vi "VIE.Module.Queued Message Handler.destroy.QueuedMessageHandler.vi"(8 "error in (no error)":errorcluster, 10 "QueuedMessageHandler.dqGOOPClass (in)":T1) -> (0 "error out":errorcluster)   [LabVIEW 2010, in "VIE.Module.Queued Message Handler.QueuedMessageHandler.dqGOOPClass.lvlib"]
uses:
  VIE.Module.Queued Message Handler.QueuedMessageHandler.dqGOOPClass.lvlib
  VIE.Module.Queued Message Handler.dqClass_ObjectReference.ctl
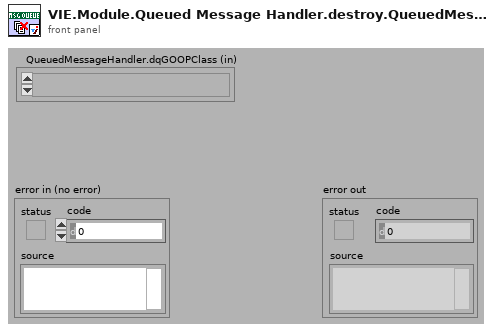
[diagram p1: front panel]
types:
  T1 = typedef "VIE.Module.Queued Message Handler.QueuedMessageHandler.dqGOOPClass.lvlib/VIE.Module.Queued Message Handler.dqClass_ObjectReference.ctl" = refnum<k1>
  T2 = typedef "VIE.Module.Queued Message Handler.QueuedMessageHandler.dqGOOPClass.lvlib/VIE.Module.Queued Message Handler.dqClass_ObjectData.ctl" = cluster{"Message Queue":refnum<queue>, "Log File Refnum":refnum<file>}
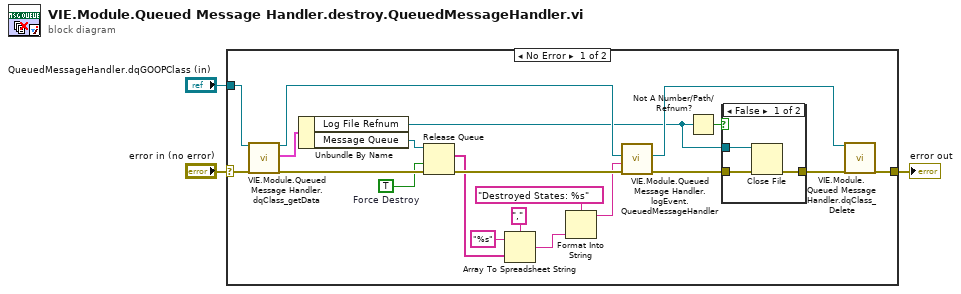
[diagram p0: block diagram]
diagram:
  n1 = case shown="No Error" "error in (no error)" {
    selector: "error in (no error)" -> [w12 w28]
    tunnel: [w15 w28] -> w2
    tunnel: "QueuedMessageHandler.dqGOOPClass (in)" -> [w9 _]
    frame No Error {
      w4 = TRUE  # Force Destroy
      n2 = call "VIE.Module.Queued Message Handler.dqClass_getData.vi"("reference"=w9, "error in (no error)"=w12) -> ("duplicate reference"=w10:T1, "data"=w11:T2, "error out"=w13:errorcluster)  [unwired: 14 in, 1 out]
      n3 = Unbundle By Name(w11) -> ("Log File Refnum"=w5:refnum<file>, "Message Queue"=w23:refnum<queue>)
      n4 = Release Queue(queue=w23, force destroy? (F)=w4, error in (no error)=w13) -> (remaining elements=w19:string[], error out=w21:errorcluster)  [unwired: 1 out]
      n5 = Array To Spreadsheet String(delimiter (Tab)=",", array=w19, 3:"%s" ("format string")) -> (spreadsheet string=w16:string)
      n6 = Format Into String(format string="Destroyed States: %s", w16) -> (resulting string=w20:string)  [unwired: 2 in, 1 out]
      n7 = call "VIE.Module.Queued Message Handler.logEvent.QueuedMessageHandler.vi"("error in (no error)"=w21, "Event to Log"=w20, "QueuedMessageHandler.dqGOOPClass (in)"=w10) -> ("error out"=w8:errorcluster, "QueuedMessageHandler.dqGOOPClass (out)"=w14:T1)  [unwired: 7 in]
      n8 = Not A Number/Path/Refnum?(number/path/refnum=w5) -> (NaN/Path/Refnum?=w6:bool)
      n9 = case shown="False" w6 {
        tunnel: w8 -> [w26 w27]
        tunnel: [w25 w27] -> w7
        tunnel: w5 -> [w24 _]
        frame False {
          n10 = Close File(refnum=w24, error in=w26) -> (error out=w25:errorcluster)  [unwired: 1 out]
        }
        frame True {
        }
      }
      n11 = call "VIE.Module.Queued Message Handler.dqClass_Delete.vi"("reference"=w14, "error in (no error)"=w7) -> ("error out"=w15:errorcluster)  [unwired: 15 in, 2 out]
    }
    frame Error {
    }
  }
  "error out" <- w2
